vi "FPGA_new_main_lock-in.vi"() -> ()   [LabVIEW 2013]
uses:
  <vilib>/eio/EIONode/EIONode.xnode
  <vilib>/rvi/DataTransferAndStorage/Container/XNode/niFpgaContainer.xnode
  <vilib>/rvi/FIFO/Fifo_Resource/nirvififoEmulationClear.vi
  <vilib>/rvi/FIFO/Fifo_Resource/nirvififoEmulationWrite.vi
  <vilib>/rvi/eio/common/nirviEmuTemplateMethod_errors.vi
  <vilib>/rvi/interface/RandomDataEmulation/nirviRandomDataFpgaReadWriteTemplate.vi
  <vilib>/rvi/FIFO/Fifo_Resource/nirvififoEmulationRead.vi
  <vilib>/rvi/Memory/Memory_Emulation/nirvimemoryFastEmulation.vi
  <vilib>/rvi/Memory/Memory_Emulation/nirvimemoryEmulation.vi
panel:
  in  "Order components":u8[](array[numeric])=[0, 0, 0, 0, 0, 0, 0, 0]
  in  "Manual order":bool
  out "get DAC value":bool
  out "moving bus":bool=TRUE
  out "order in":u64
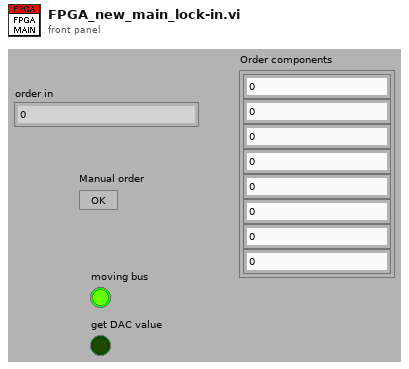
[diagram p1: front panel]
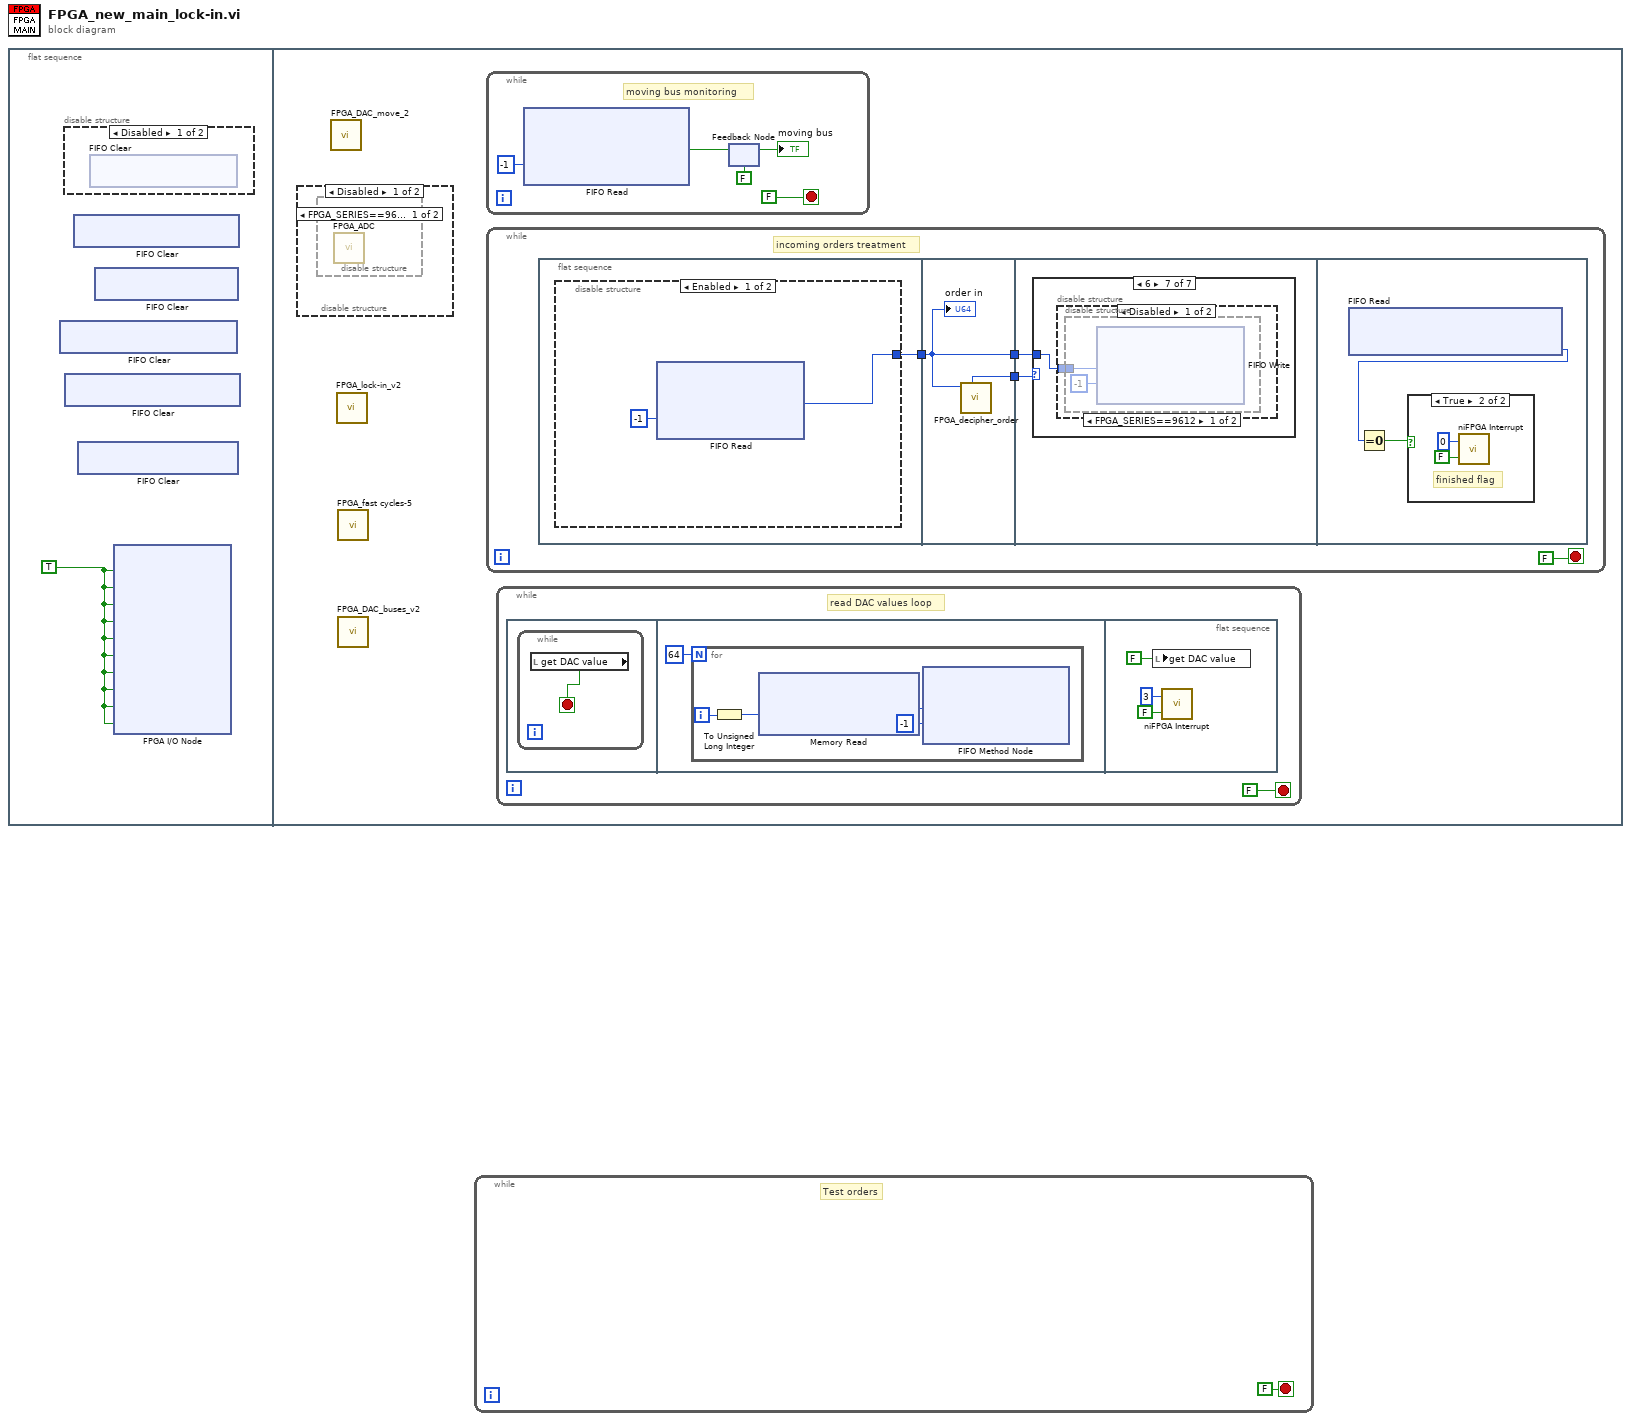
[diagram p0: block diagram]
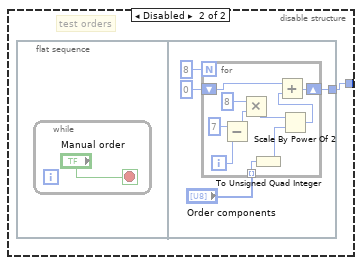
[diagram p5: hidden frame]
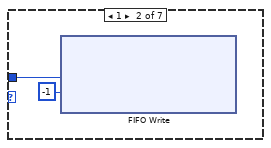
[diagram p7: hidden frame]
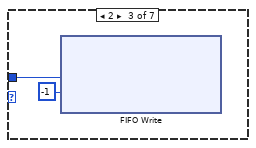
[diagram p8: hidden frame]
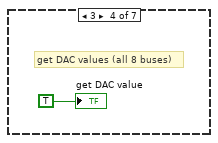
[diagram p9: hidden frame]
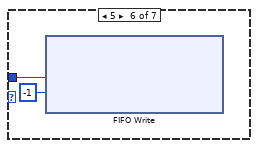
[diagram p11: hidden frame]
diagram:
  n1 = flat-sequence {
    frame #0 {
      w1 = TRUE ("Port0/DIOCTL")
      n2 = xnode ("FIFO Clear")() -> ()  [unwired: 1 in, 1 out]
      n3 = disable-structure shown="Disabled" {
        frame Disabled {
          n4 = xnode ("FIFO Clear")() -> ()  [unwired: 1 in, 1 out]
        }
        frame Enabled {
        }
      }
      n5 = xnode ("FIFO Clear")() -> ()  [unwired: 1 in, 1 out]
      n6 = xnode ("FIFO Clear")() -> ()  [unwired: 1 in, 1 out]
      n7 = xnode ("FIFO Clear")() -> ()  [unwired: 1 in, 1 out]
      n8 = xnode ("FIFO Clear")() -> ()  [unwired: 1 in, 1 out]
      n9 = xnode "FPGA I/O Node"("Port0/DIOCTL"=w1, "Port1/DIOCTL"=w1, "Port2/DIOCTL"=w1, "Port3/DIOCTL"=w1, "Port4/DIOCTL"=w1, "Port5/DIOCTL"=w1, "Port6/DIOCTL"=w1, "Port7/DIOCTL"=w1, "Port8/DIOCTL"=w1, "Port9/DIOCTL"=w1) -> ()  [unwired: 10 in, 10 out]
    }
    frame #1 {
      n10 = disable-structure shown="Disabled" {
        frame Disabled {
          n11 = disable-structure shown="FPGA_SERIES==9612" {
            frame condition #0 {
              n12 = call "FPGA_ADC.vi"() -> ()  [unwired: 12 in]
            }
            frame condition #1 (active) {
            }
          }
        }
        frame Enabled {
        }
      }
      n13 = call "FPGA_DAC_move_2.vi"() -> ()  [unwired: 3 in]
      n14 = call "FPGA_lock-in_v2.vi"() -> ()  [unwired: 1 in]
      n15 = call "FPGA_fast cycles-5.vi"() -> ()  [unwired: 1 in]
      n16 = call "FPGA_DAC_buses_v2.vi"() -> ()  [unwired: 12 in]
      n17 = while {
        stop <- FALSE stop-if-true
        # "moving bus monitoring"
        n18 = xnode ("FIFO Read")("Timeout"=-1) -> ("Element"=w12:bool)  [unwired: 1 in, 2 out]
        n19 = feedback-in #1(w12) -> ()
        n20 = feedback #1(FALSE ("Element")) -> (→"moving bus":bool)
      }
      n21 = while {
        stop <- FALSE stop-if-true
        # "incoming orders treatment"
        n22 = flat-sequence {
          tunnel: [w21] -> w17
          tunnel: [w40] -> w19
          tunnel: [w41] -> w18
          tunnel: w17 -> [w40]
          tunnel: w19 -> [w43]
          tunnel: w18 -> [w42]
          frame #0 {
            n23 = disable-structure shown="Enabled" {
              disable-tunnel: [w22 w24] -> w21
              frame Enabled {
                n24 = xnode ("FIFO Read")("Timeout"=-1) -> ("Element"=w22:u64)  [unwired: 1 in, 2 out]
              }
              frame Disabled {
                # "test orders"
                n25 = flat-sequence {
                  tunnel: [w26] -> w24
                  frame #0 {
                    n26 = while {
                      stop <- "Manual order" stop-if-true
                    }
                  }
                  frame #1 {
                    n27 = for {
                      N: 8 -> [_]
                      tunnel: "Order components" -> [w34] mode=indexing
                      shift-right: [w33] -> w26
                      shift-left: u64 0 -> [w32]
                      i -> [w38]
                      n28 = Subtract(x=7, y=w38) -> (x-y=w37:i32)
                      n29 = Multiply(x=8, y=w37) -> (x*y=w35:i32)
                      n30 = To Unsigned Quad Integer(1:w34) -> (0:w31:u64)
                      n31 = Scale By Power Of 2(n=w35, x=w31) -> (x*2^n=w30:u64)
                      n32 = Add(x=w32, y=w30) -> (x+y=w33:u64)
                    }
                  }
                }
              }
            }
          }
          frame #1 {
            n33 = call "FPGA_decipher_order.vi"("order in"=w40) -> ("subsystem"=w41:u8)  [unwired: 10 out]
            "order in" <- w40
          }
          frame #2 {
            n34 = case shown="6" w42 {
              tunnel: w43 -> [_ w44 w46 _ _ w49 w51]
              frame 0, Default {
              }
              frame 1 {
                n35 = xnode ("FIFO Write")("Element"=w44, "Timeout"=-1) -> ()  [unwired: 1 in, 2 out]
              }
              frame 2 {
                n36 = xnode ("FIFO Write")("Element"=w46, "Timeout"=-1) -> ()  [unwired: 1 in, 2 out]
              }
              frame 3 {
                # "get DAC values (all 8 buses)"
                "get DAC value" <- TRUE ("get DAC values")
              }
              frame 4 {
                # "removed"
              }
              frame 5 {
                n37 = xnode ("FIFO Write")("Element"=w49, "Timeout"=-1) -> ()  [unwired: 1 in, 2 out]
              }
              frame 6 {
                n38 = disable-structure shown="Disabled" {
                  disable-tunnel: w51 -> [w52 _]
                  frame Disabled {
                    n39 = disable-structure shown="FPGA_SERIES==9612" {
                      disable-tunnel: w52 -> [w54 _]
                      frame condition #0 {
                        n40 = xnode ("FIFO Write")("Element"=w54, "Timeout"=-1) -> ()  [unwired: 1 in, 2 out]
                      }
                      frame condition #1 (active) {
                      }
                    }
                  }
                  frame Enabled {
                  }
                }
              }
            }
          }
          frame #3 {
            n41 = xnode ("FIFO Read")() -> ("Number of Elements to Read"=w55:u32)  [unwired: 1 in, 1 out]
            n42 = Equal To 0?(x=w55) -> (x = 0?=w56:bool)
            n43 = case shown="True" w56 {
              frame False {
              }
              frame True {
                # "finished flag"
                n44 = call <vilib>:"niFPGA Interrupt.vi"("Wait Until Cleared (F)"=FALSE, "IRQ Number (0)"=u8 0) -> ()  [unwired: 1 in]
              }
            }
          }
        }
      }
      n45 = while {
        stop <- FALSE stop-if-true
        # "read DAC values loop"
        n46 = flat-sequence {
          frame #0 {
            n47 = while {
              stop <- w3 stop-if-true
              n48 = local read "get DAC value"() -> (w3:bool)
            }
          }
          frame #1 {
            n49 = for {
              N: 64 -> [_]
              i -> [w7]
              n50 = To Unsigned Long Integer(number=w7) -> (unsigned 32bit integer=w8:u32)
              n51 = xnode ("Memory Read")("Address"=w8) -> ("Data"=w6:u16)  [unwired: 1 in, 1 out]
              n52 = xnode ("FIFO Method Node")("Element"=w6, "Timeout"=-1) -> ()  [unwired: 1 in, 2 out]
            }
          }
          frame #2 {
            n53 = local write "get DAC value"(FALSE ("get DAC values")) -> ()
            n54 = call <vilib>:"niFPGA Interrupt.vi"("Wait Until Cleared (F)"=FALSE, "IRQ Number (0)"=u8 3) -> ()  [unwired: 1 in]
          }
        }
      }
    }
  }
  n55 = while {
    stop <- FALSE stop-if-true
    # "Test orders"
  }
